vi "B020上传.vi"(2 "数据":string[](array[string])) -> ()   [LabVIEW 2013]
uses:
  <vilib>/Utility/error.llb/whitespace.ctl
panel:
  out "连接的字符串":string
  in  "数据名":string[](array[string])
  in  "error in (no error)":errorcluster
  out "error out":errorcluster
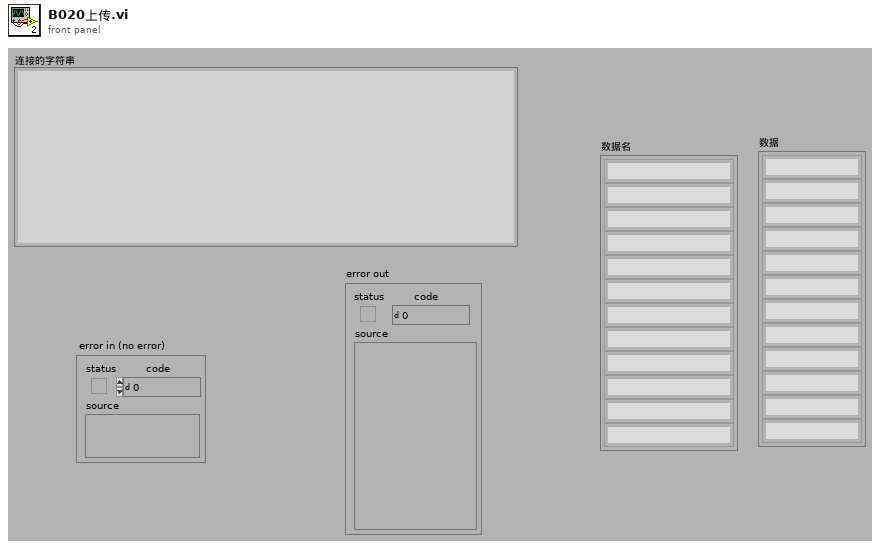
[diagram p1: front panel]
types:
  T1 = typedef "whitespace.ctl" = u16
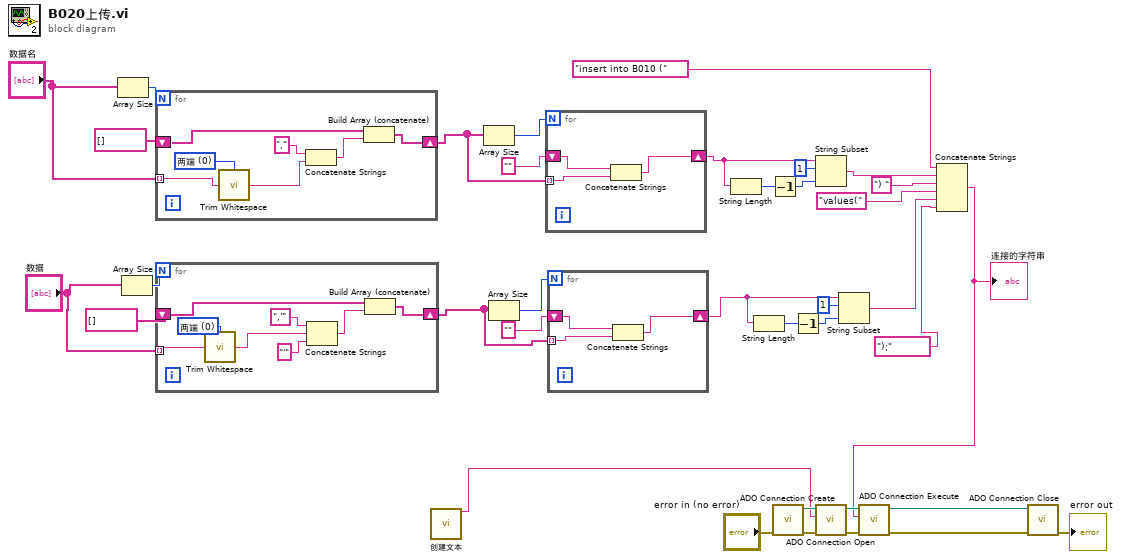
[diagram p0: block diagram]
diagram:
  n1 = Array Size(array="数据名") -> (size(s)=w27:i32)
  n2 = Array Size(array="数据") -> (size(s)=w14:i32)
  n3 = for {
    N: w27 -> [_]
    tunnel: "数据名" -> [w39] mode=indexing
    shift-right: [w42] -> w22
    shift-left: string[] [] ("添加的数组") -> [w41]
    w38 = T1 0 items=["两端", "字符串首端", "字符串末端"] ("location (both)")
    n4 = call <vilib>:"Trim Whitespace.vi"("string"=w39, "location (both)"=w38) -> ("trimmed string"=w37:string)
    n5 = Concatenate Strings("," ("字符串"), w37) -> (w43:string)
    n6 = Build Array (concatenate)(w41, w43) -> (w42:string[])
  }
  n7 = for {
    N: w14 -> [_]
    tunnel: "数据" -> [w46] mode=indexing
    shift-right: [w50] -> w9
    shift-left: string[] [] ("添加的数组") -> [w49]
    w45 = T1 0 items=["两端", "字符串首端", "字符串末端"] ("location (both)")
    n8 = call <vilib>:"Trim Whitespace.vi"("string"=w46, "location (both)"=w45) -> ("trimmed string"=w44:string)
    n9 = Concatenate Strings(",'" ("字符串"), w44, "'" ("字符串")) -> (w51:string)
    n10 = Build Array (concatenate)(w49, w51) -> (w50:string[])
  }
  n11 = call "创建文本"() -> ("Result"=w28:string)  [unwired: 14 in, 1 out]
  n12 = Array Size(array=w22) -> (size(s)=w23:i32)
  n13 = Array Size(array=w9) -> (size(s)=w11:i32)
  n14 = for {
    N: w23 -> [_]
    tunnel: w22 -> [w54] mode=indexing
    shift-right: [w52] -> w20
    shift-left: "" -> [w53]
    n15 = Concatenate Strings(w53, w54) -> (w52:string)
  }
  n16 = for {
    N: w11 -> [_]
    tunnel: w9 -> [w57] mode=indexing
    shift-right: [w55] -> w6
    shift-left: "" -> [w56]
    n17 = Concatenate Strings(w56, w57) -> (w55:string)
  }
  n18 = String Length(string=w20) -> (length=w19:i32)
  n19 = String Length(string=w6) -> (length=w7:i32)
  n20 = Decrement(x=w19) -> (x-1=w18:i32)
  n21 = call "ADO Connection Create.vi"("error in (no error)"="error in (no error)") -> ("error out"=w35:errorcluster, "ADODB._Connection Out"=w36:refnum<k7>)  [unwired: 9 out]
  n22 = Decrement(x=w7) -> (x-1=w8:i32)
  n23 = String Subset(string=w20, offset (0)=1 ("偏移量(0)"), length (rest)=w18) -> (substring=w17:string)
  n24 = call "ADO Connection Open.vi"("error in (no error)"=w35, "ConnectionString"=w28, "ADODB._Connection In"=w36) -> ("error out"=w34:errorcluster, "ADODB._Connection Out"=w33:refnum<k7>)  [unwired: 7 out]
  n25 = String Subset(string=w6, offset (0)=1 ("偏移量(0)"), length (rest)=w8) -> (substring=w5:string)
  n26 = Concatenate Strings("insert into B010 (" ("字符串"), w17, ") " ("字符串"), "values(" ("字符串"), w5, ");" ("字符串")) -> (w3:string)
  "连接的字符串" <- w3
  n27 = call "ADO Connection Execute.vi"("error in (no error)"=w34, "CommandText"=w3, "ADODB._Connection In"=w33) -> ("error out"=w29:errorcluster, "ADODB._Connection Out"=w32:refnum<k7>)  [unwired: 7 out]
  n28 = call "ADO Connection Close.vi"("error in (no error)"=w29, "ADODB._Connection In"=w32) -> ("error out"=→"error out":errorcluster)  [unwired: 9 out]
